vi "DE_Perturb Scale Factor.vi"(10 "number of parameters":i32, 11 "scale factor":dbl) -> (3 "Perturbed Scale Factors":dbl[](array[numeric]))   [LabVIEW 2017, in "NI_AAL_GlobalOptimization.lvlib"]
uses:
  <vilib>/gmath/NI_AAL_GlobalOptimization.lvlib
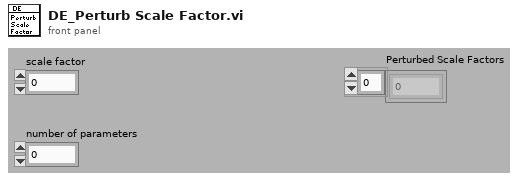
[diagram p1: front panel]
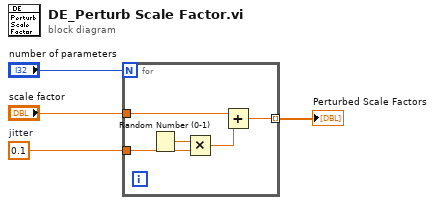
[diagram p0: block diagram]
diagram:
  w1 = 0.1  # jitter
  n1 = for {
    N: "number of parameters" -> [_]
    tunnel: "scale factor" -> [w6]
    tunnel: [w7] -> w2 mode=indexing
    tunnel: w1 -> [w5]
    n2 = Random Number (0-1)() -> (number: 0 to 1=w9:dbl)
    n3 = Multiply(x=w9, y=w5) -> (x*y=w8:dbl)
    n4 = Add(x=w6, y=w8) -> (x+y=w7:dbl)
  }
  "Perturbed Scale Factors" <- w2
